vi "PlotTve.vi"(8 "ErrorArray":errorcluster[](array[cluster]), 9 "TvePlotRef":refnum<vi>, 10 "clPMUImpairRptArray":T1 {"Synx" format="%#_4g"}, 11 "clEvtReportArray":T1 {"Synx" format="%#_4g"}) -> (0 "ErrorArray":errorcluster[](array[cluster]))   [LabVIEW 2017, in "Visualization.lvlib" / "VisualizePMU_class.lvclass"]
uses:
  VisualizePMU_class.lvclass
  Modules/EventPlugins/EventPluginBaseClass/TypeDefs/clEvtReportArray.ctl
  Modules/EventPlugins/EventPluginBaseClass/TypeDefs/clEvtReport.ctl
  <userlib>/NIST/NISTErrorLib/NISTErrorLib.lvlib
  Modules/EventPlugins/EventPluginBaseClass/EventPluginBaseClass.lvclass
panel:
  out "TVE Plot":cluster{dbl[], "TVE":dbl[]}[](graph)
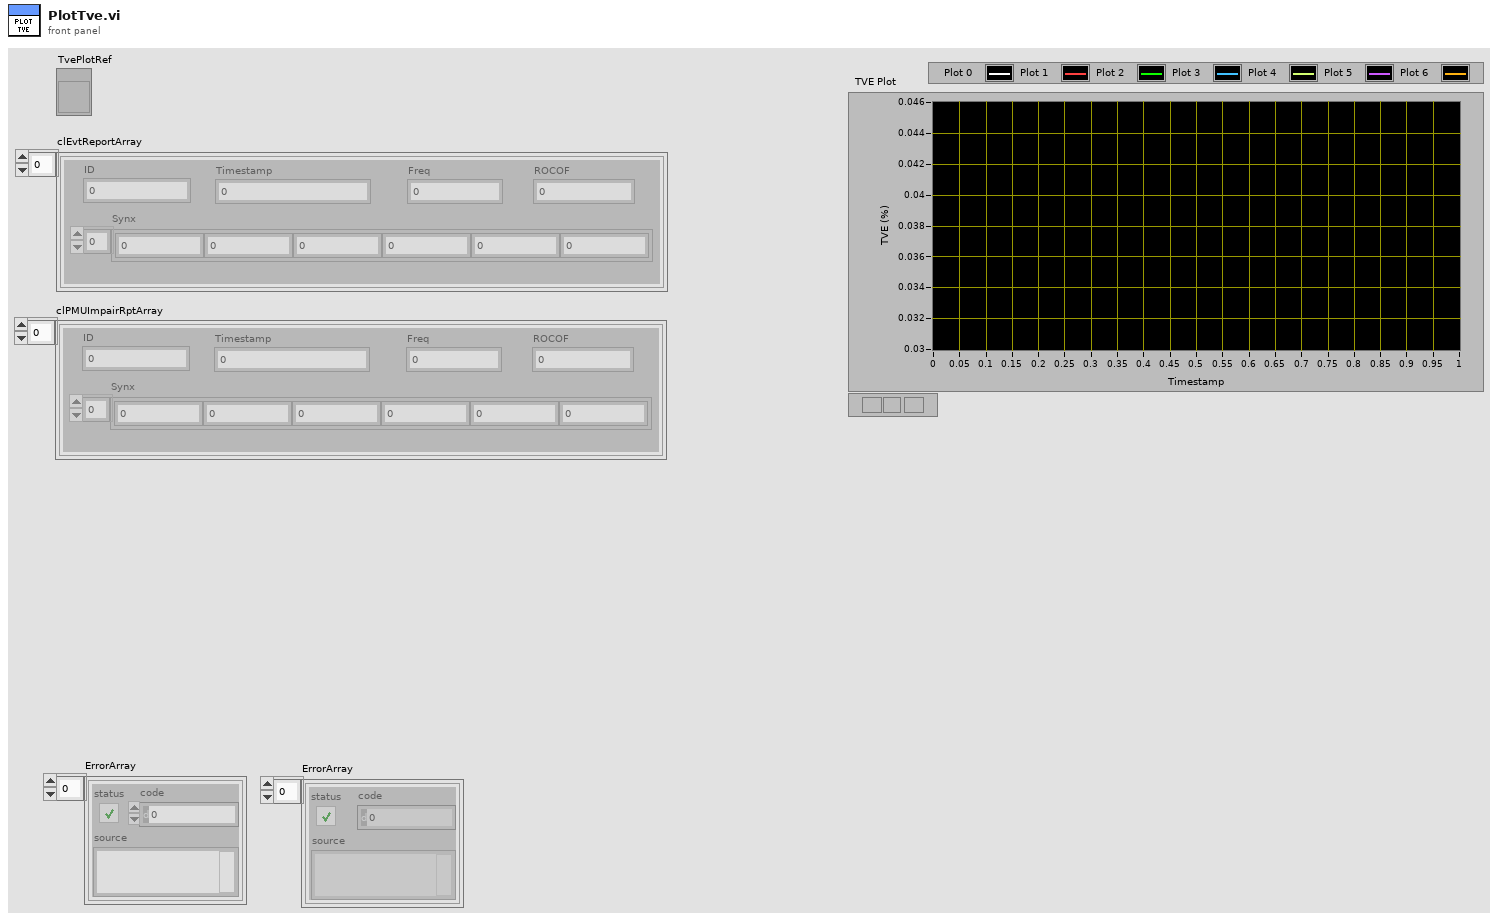
[diagram p1: front panel]
types:
  T1 = typedef "EventPlugins.lvlib/EventPluginBaseClass.lvclass/clEvtReportArray.ctl" = T2[]
  T2 = typedef "EventPlugins.lvlib/EventPluginBaseClass.lvclass/clEvtReport.ctl" = cluster{"Timestamp":dbl, "Synx":cdb[], "Freq":dbl, "ROCOF":dbl, "ID":i16}
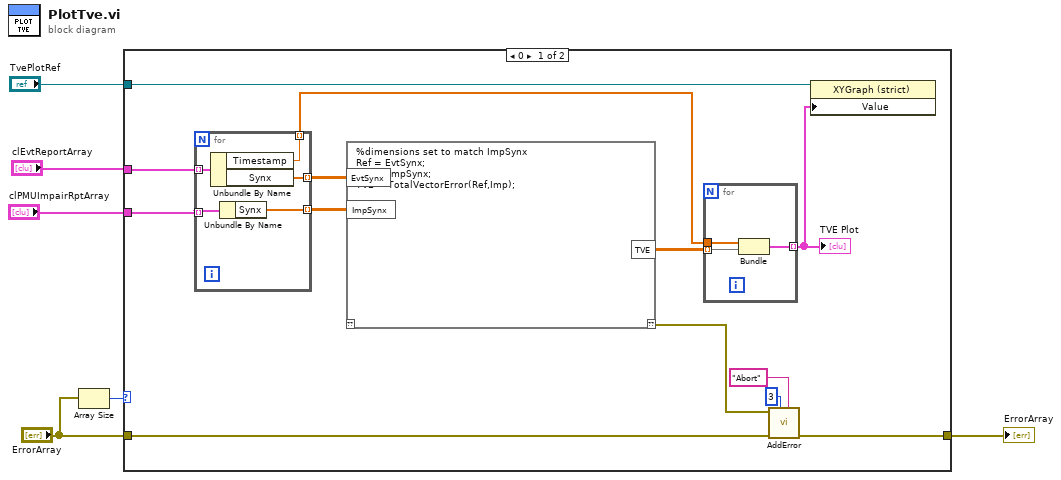
[diagram p0: block diagram]
diagram:
  n1 = Array Size(array="ErrorArray") -> (size(s)=w6:i32)
  n2 = case shown="0" w6 {
    tunnel: "ErrorArray" -> [w9 w28]
    tunnel: [w13 w28] -> w4
    tunnel: "clEvtReportArray" -> [w19 _]
    tunnel: "clPMUImpairRptArray" -> [w18 _]
    tunnel: "TvePlotRef" -> [w8 _]
    frame 0 {
      n3 = for {
        tunnel: w18 -> [w27] mode=indexing
        tunnel: w19 -> [w26] mode=indexing
        tunnel: [w25] -> w17 mode=indexing
        tunnel: [w24] -> w16 mode=indexing
        tunnel: [w23] -> w14 mode=indexing
        n4 = Unbundle By Name(w26) -> ("Timestamp"=w23:dbl, "Synx"=w25:cdb[])
        n5 = Unbundle By Name(w27) -> ("Synx"=w24:cdb[])
      }
      n6 = script code="%dimensions set to match ImpSynx\nRef = EvtSynx;\nImp = ImpSynx;\nTVE = TotalVectorError(Ref,Imp);"("EvtSynx"=w17, "ImpSynx"=w16) -> ("??"=w12:errorcluster, "TVE"=w15:dbl[][])  [unwired: 1 in]
      n7 = for {
        tunnel: w15 -> [w22] mode=indexing
        tunnel: w14 -> [w21]
        tunnel: [w20] -> w7 mode=indexing
        n8 = Bundle(w21, w22) -> (w20:cluster{dbl[], dbl[]})  [unwired: 1 in]
      }
      "TVE Plot" <- w7
      n9 = call <userlib>:"AddError.vi"("Severity"="Abort" ("String"), "Priority"=u8 3, "ErrorArray"=w9, "error in (no error)"=w12) -> ("ErrorArray"=w13:errorcluster[])  [unwired: 6 in, 1 out]
      n10 = property class="XYGraph (strict)"(reference=w8, "Value"=w7) -> ()  [unwired: 1 in, 2 out]
    }
    frame 1, Default {
    }
  }
  "ErrorArray" <- w4
